vi "Set_Unit.vi"(2 "error in":errorcluster, 3 "Unit":string(combo), 4 "VISA arduino in":refnum<visa-resource-name>) -> (0 "error out":errorcluster, 1 "VISA arduino out":refnum<visa-resource-name>)   [LabVIEW 2021]
uses:
  <vilib>/Utility/error.llb/Error Cluster From Error Code.vi
  <vilib>/ErrorRing/Error Ring.xnode
panel:
  out "delay":u32
  # "Private"
  # "Public"
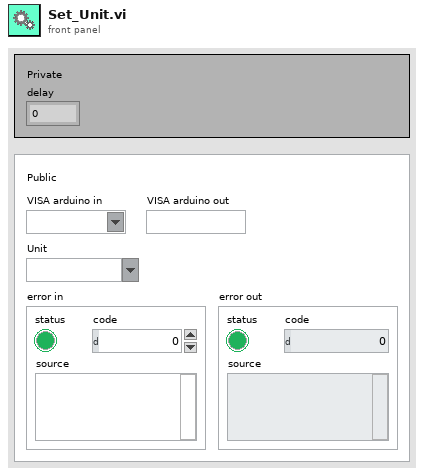
[diagram p1: front panel]
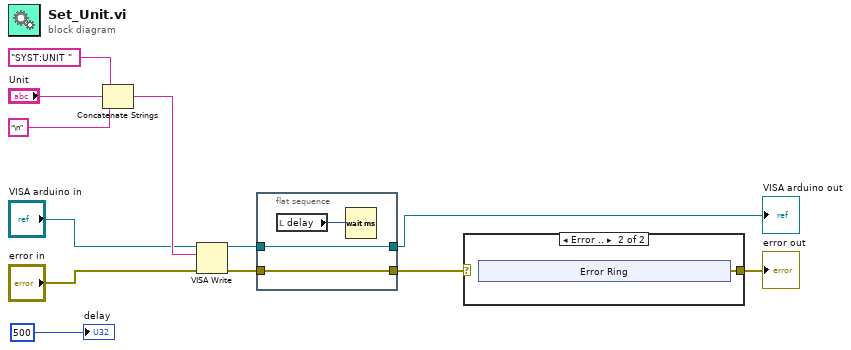
[diagram p0: block diagram]
diagram:
  n1 = Concatenate Strings("SYST:UNIT ", "Unit", "\n" ("string")) -> (w3:string)
  n2 = VISA Write(VISA resource name="VISA arduino in", write buffer=w3, error in (no error)="error in") -> (VISA resource name out=w10:refnum<visa-resource-name>, error out=w9:errorcluster)  [unwired: 1 out]
  n3 = flat-sequence {
    tunnel: [w15] -> w6
    tunnel: w10 -> [w15]
    tunnel: [w14] -> w11
    tunnel: w9 -> [w14]
    frame #0 {
      n4 = local read "delay"() -> (w13:u32)
      n5 = Wait (ms)(milliseconds to wait=w13) -> ()  [unwired: 1 out]
    }
  }
  n6 = case shown="Error .." w11 {
    selector: w11 -> [w16 _]
    tunnel: [w16 w17] -> w7
    frame No Error {
    }
    frame Error {
      n7 = xnode "Error Ring"() -> ("error out"=w17:errorcluster)
    }
  }
  "error out" <- w7
  "delay" <- u32 500
  "VISA arduino out" <- w6
